vi "unique-name-differnetowner-test.vi"(8 "error in (no error)":errorcluster) -> (0 "error out":errorcluster)   [LabVIEW 2013]
uses:
  src/SMO/SMO.lvclass
  <vilib>/addons/_JKI Toolkits/Caraya/classes/Test/Test.lvclass
  <vilib>/addons/_JKI Toolkits/Caraya/classes/Assert/Assert.lvclass
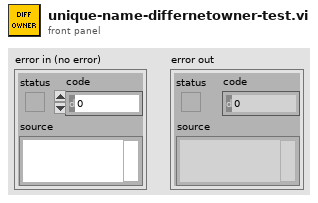
[diagram p1: front panel]
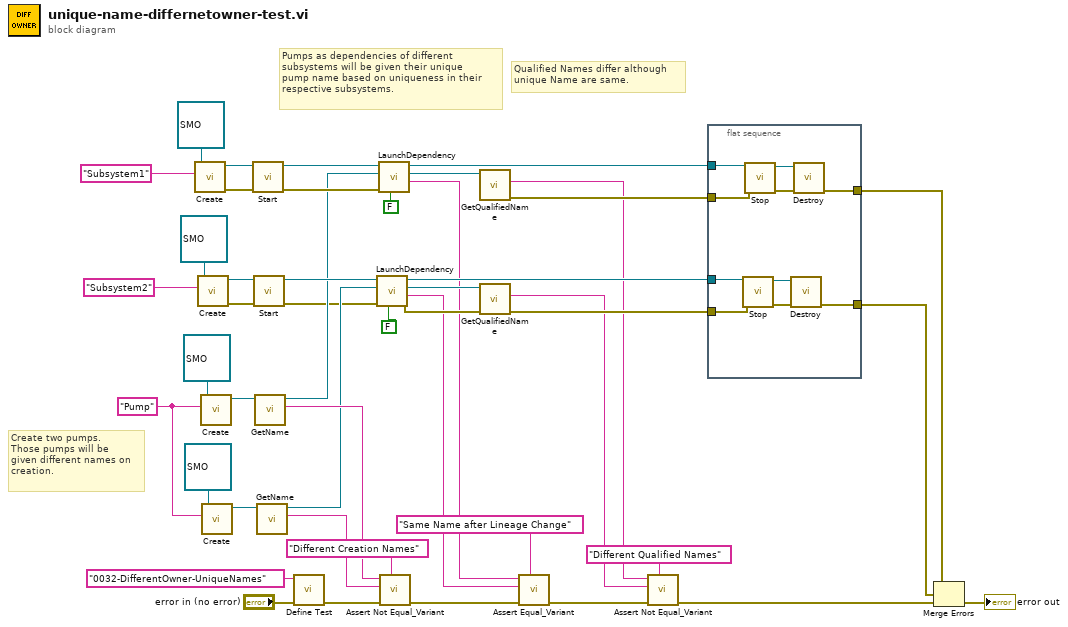
[diagram p0: block diagram]
diagram:
  w1 = "Pump" ("Subsystem Name (optional)")
  # "Qualified Names differ although\nunique Name are same."
  # "Pumps as dependencies of different\nsubsystems will be given their unique\npump name based on uniqueness in their\nrespective subsystems."
  # "Create two pumps.\nThose pumps will be\ngiven different names on\ncreation."
  n1 = call "Create.vi"("Subsystem Name (optional)"="Subsystem1", "SMO"=refnum<class "SMO.lvclass"> refnum ("SMO.lvclass")) -> ("error out"=w39:errorcluster, "SMO out"=w40:refnum<class "SMO.lvclass">)  [unwired: 7 in, 1 out]
  n2 = call "Create.vi"("Subsystem Name (optional)"="Subsystem2", "SMO"=refnum<class "SMO.lvclass"> refnum ("SMO.lvclass")) -> ("error out"=w38:errorcluster, "SMO out"=w37:refnum<class "SMO.lvclass">)  [unwired: 7 in, 1 out]
  n3 = call "Create.vi"("Subsystem Name (optional)"=w1, "SMO"=refnum<class "SMO.lvclass"> refnum ("SMO.lvclass")) -> ("SMO out"=w8:refnum<class "SMO.lvclass">)  [unwired: 7 in, 2 out]
  n4 = call "Create.vi"("Subsystem Name (optional)"=w1, "SMO"=refnum<class "SMO.lvclass"> refnum ("SMO.lvclass")) -> ("SMO out"=w5:refnum<class "SMO.lvclass">)  [unwired: 7 in, 2 out]
  n5 = call "Start.vi"("error in (no error)"=w39, "SMO"=w40) -> ("error out"=w35:errorcluster, "SMO out"=w36:refnum<class "SMO.lvclass">)  [unwired: 8 in]
  n6 = call "Start.vi"("error in (no error)"=w38, "SMO"=w37) -> ("error out"=w2:errorcluster, "SMO out"=w34:refnum<class "SMO.lvclass">)  [unwired: 8 in]
  n7 = call "GetName.vi"("SMO"=w8) -> ("Name"=w6:string, "SMO out"=w7:refnum<class "SMO.lvclass">)  [unwired: 7 in, 2 out]
  n8 = call "GetName.vi"("SMO"=w5) -> ("Name"=w3:string, "SMO out"=w4:refnum<class "SMO.lvclass">)  [unwired: 7 in, 2 out]
  n9 = call <vilib>:"Define Test.vi"("error in (no error)"="error in (no error)", "Label (VI Title)"="0032-DifferentOwner-UniqueNames") -> ("error out"=w11:errorcluster)  [unwired: 9 in]
  n10 = call "LaunchDependency.vi"("Shared Resource"=FALSE, "error in (no error)"=w2, "Dependency Type"=w4, "SMO in"=w34) -> ("error out"=w29:errorcluster, "Unique Name"=w21:string, "Dependency Reference"=w30:refnum<class "SMO.lvclass">, "SMO out"=w26:refnum<class "SMO.lvclass">)  [unwired: 4 in]
  n11 = call "LaunchDependency.vi"("Shared Resource"=FALSE, "error in (no error)"=w35, "Dependency Type"=w7, "SMO in"=w36) -> ("Unique Name"=w22:string, "Dependency Reference"=w31:refnum<class "SMO.lvclass">, "SMO out"=w28:refnum<class "SMO.lvclass">)  [unwired: 4 in, 1 out]
  n12 = call <vilib>:"Assert Not Equal_Variant.vi"("Label"="Different Creation Names", "error in (no error)"=w11, "Y"=w3, "X"=w6) -> ("error out"=w10:errorcluster)  [unwired: 7 in]
  n13 = call "GetQualifiedName.vi"("SMO"=w31) -> ("error out"=w27:errorcluster, "Qualified Name"=w16:string)  [unwired: 8 in, 1 out]
  n14 = call "GetQualifiedName.vi"("error in (no error)"=w29, "SMO"=w30) -> ("error out"=w25:errorcluster, "Qualified Name"=w15:string)  [unwired: 7 in, 1 out]
  n15 = call <vilib>:"Assert Equal_Variant.vi"("Label"="Same Name after Lineage Change", "error in (no error)"=w10, "Y"=w21, "X"=w22) -> ("error out"=w18:errorcluster)  [unwired: 7 in]
  n16 = call <vilib>:"Assert Not Equal_Variant.vi"("Label"="Different Qualified Names", "error in (no error)"=w18, "Y"=w15, "X"=w16) -> ("error out"=w17:errorcluster)  [unwired: 7 in]
  n17 = flat-sequence {
    tunnel: [w48] -> w24
    tunnel: [w47] -> w23
    tunnel: w28 -> [w56]
    tunnel: w27 -> [w55]
    tunnel: w26 -> [w54]
    tunnel: w25 -> [w53]
    frame #0 {
      n18 = call "Stop.vi"("error in (no error)"=w53, "SMO"=w54) -> ("error out"=w50:errorcluster, "SMO out"=w49:refnum<class "SMO.lvclass">)  [unwired: 8 in]
      n19 = call "Stop.vi"("error in (no error)"=w55, "SMO"=w56) -> ("error out"=w52:errorcluster, "SMO out"=w51:refnum<class "SMO.lvclass">)  [unwired: 8 in]
      n20 = call "Destroy.vi"("error in (no error)"=w50, "SMO"=w49) -> ("error out"=w47:errorcluster)  [unwired: 9 in]
      n21 = call "Destroy.vi"("error in (no error)"=w52, "SMO"=w51) -> ("error out"=w48:errorcluster)  [unwired: 9 in]
    }
  }
  n22 = Merge Errors(w24, w23, w17) -> (→"error out":errorcluster)
